vi "Initialize.vi"(8 "error in (no error)":errorcluster, 11 "ChromaPowerSupply in":refnum<class "ChromaPowerSupply.lvclass">) -> (0 "error out":errorcluster, 3 "ChromaPowerSupply out":refnum<class "ChromaPowerSupply.lvclass">)   [LabVIEW 2018, in "AcPwrPlugins.lvlib" / "ChromaPowerSupply.lvclass"]
doc: "This VI establishes communication to the instrument and may provide other functions such as reset the instrument or provide a range check."
uses:
  ChromaPowerSupply.lvclass
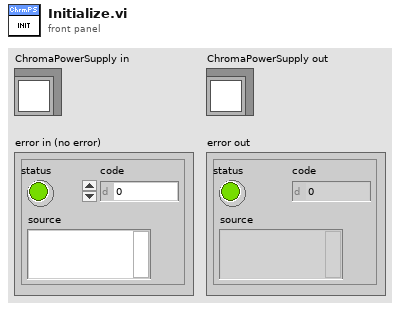
[diagram p1: front panel]
types:
  T1 = cluster{"Handle Connected?":bool, "instrument handle out":refnum<k15>}[]
  T2 = typedef "AcPwrPlugins.lvlib/ChromaPowerSupply.lvclass/Measurements.ctl" = cluster{"Handle":string, "Name":string, "Enabled":bool, "Measurement Value":dbl, "btnMeasFetch":bool, "ProtectionStatusString":string, "Measurement Type":enum16{"Voltage", "Current", "Power"}}[]
  T3 = typedef "AcPwrPlugins.lvlib/ChromaPowerSupply.lvclass/Device(s)Settings.ctl" = cluster{"Phases":cluster{"Handle":string, "Instrument Options":string, "id query (T)":bool, "reset device (T)":bool, "Timing":cluster{"TimingOn":enum16{""}, "Hours":u32, "Minutes":u32, "Seconds":dbl, "CutoffVoltage":dbl}, "Connected":bool, "Output Mode":enum16{"Voltage (DC)", "Current (DC)"}, "Voltage":dbl, "Current":dbl, "High Voltage Limit":dbl, "High Current Limit":dbl, "Power Protect":dbl, "Current Protect":dbl, "Voltage Protect":dbl, "Low Current Limit":dbl, "Low Voltage Limit":dbl, "Current Slew Rate":dbl, "Voltage Slew Rate":dbl, "Current Slew Infinite?":bool}[], "MeasName":string}
  T4 = cluster{"Handle":string, "Instrument Options":string, "id query (T)":bool, "reset device (T)":bool, "Timing":cluster{"TimingOn":enum16{""}, "Hours":u32, "Minutes":u32, "Seconds":dbl, "CutoffVoltage":dbl}, "Connected":bool, "Output Mode":enum16{"Voltage (DC)", "Current (DC)"}, "Voltage":dbl, "Current":dbl, "High Voltage Limit":dbl, "High Current Limit":dbl, "Power Protect":dbl, "Current Protect":dbl, "Voltage Protect":dbl, "Low Current Limit":dbl, "Low Voltage Limit":dbl, "Current Slew Rate":dbl, "Voltage Slew Rate":dbl, "Current Slew Infinite?":bool}[]
  T5 = cluster{"Handle Connected?":bool, "instrument handle out":refnum<k15>}
  T6 = cluster{"Handle":string, "Instrument Options":string, "id query (T)":bool, "reset device (T)":bool, "Timing":cluster{"TimingOn":enum16{""}, "Hours":u32, "Minutes":u32, "Seconds":dbl, "CutoffVoltage":dbl}, "Connected":bool, "Output Mode":enum16{"Voltage (DC)", "Current (DC)"}, "Voltage":dbl, "Current":dbl, "High Voltage Limit":dbl, "High Current Limit":dbl, "Power Protect":dbl, "Current Protect":dbl, "Voltage Protect":dbl, "Low Current Limit":dbl, "Low Voltage Limit":dbl, "Current Slew Rate":dbl, "Voltage Slew Rate":dbl, "Current Slew Infinite?":bool}
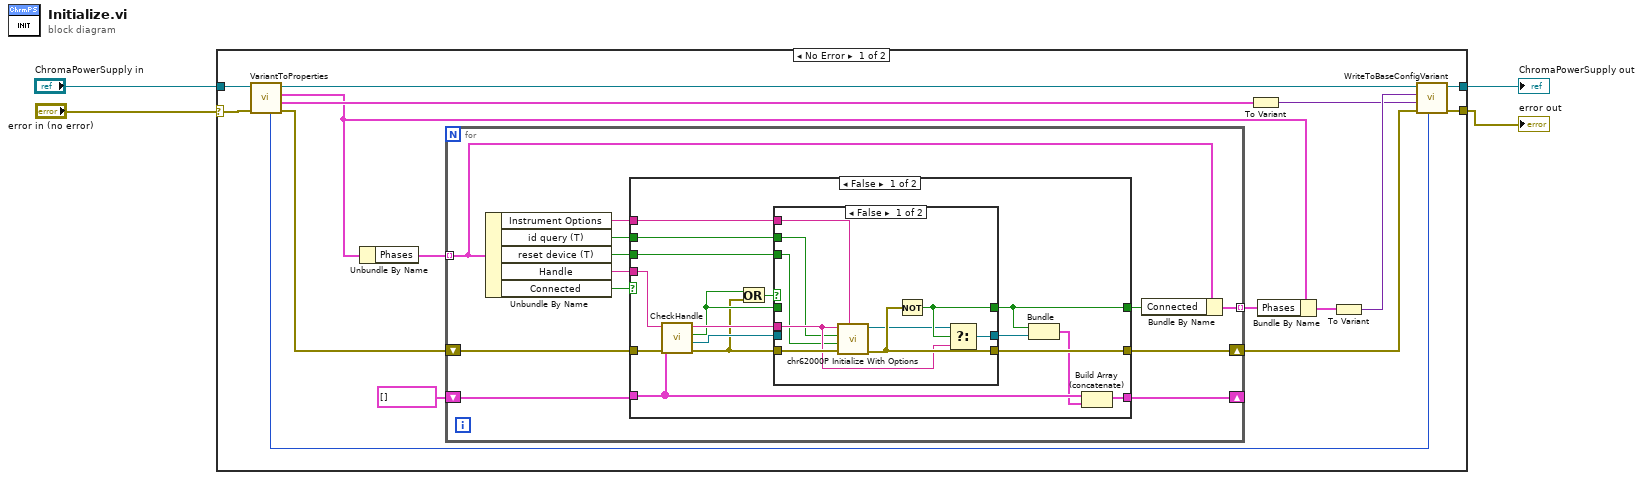
[diagram p0: block diagram]
diagram:
  n1 = case shown="No Error" "error in (no error)" {
    selector: "error in (no error)" -> [w20 w65]
    tunnel: "ChromaPowerSupply in" -> [w10 w64]
    tunnel: [w17 w64] -> w2
    tunnel: [w16 w65] -> w1
    frame No Error {
      n2 = call-dynamic "VariantToProperties.vi"("error in (no error)"=w20, "ChromaPowerSupply in"=w10) -> ("error out"=w19:errorcluster, "Measurements"=w12:T2, "Device Settings"=w7:T3, "ChromaPowerSupply out"=w14:refnum<class "ChromaPowerSupply.lvclass">, "Measurement Refresh Time (ms)"=w11:u32)  [unwired: 5 in]
      n3 = Unbundle By Name(w7) -> ("Phases"=w9:T4)
      n4 = for {
        tunnel: w9 -> [w22] mode=indexing
        shift-right: [w30] -> w15
        shift-left: w19 -> [w31]
        shift-right: [w23] -> _
        shift-left: T1 [] -> [w32]
        tunnel: [w21] -> w8 mode=indexing
        n5 = Unbundle By Name(w22) -> ("Instrument Options"=w26:string, "id query (T)"=w25:bool, "reset device (T)"=w24:bool, "Handle"=w29:string, "Connected"=w28:bool)
        n6 = case shown="False" w28 {
          selector: w28 -> [_ w63]
          tunnel: [w43 w63] -> w27
          tunnel: w29 -> [w48 _]
          tunnel: [w44 w62] -> w30
          tunnel: w31 -> [w37 w62]
          tunnel: w32 -> [w34 w61]
          tunnel: [w46 w61] -> w23
          tunnel: w26 -> [w42 _]
          tunnel: w25 -> [w41 _]
          tunnel: w24 -> [w40 _]
          frame False {
            n7 = call "CheckHandle.vi"("error in (no error)"=w37, "Array"=w34, "Handle In"=w48) -> ("error out"=w35:errorcluster, "instrument handle out"=w39:refnum<k15>, "Handle Connected?"=w36:bool, "Handle Out"=w38:string)  [unwired: 5 in]
            n8 = Or(x=w36, y=w35) -> (x .or. y?=w47:bool)
            n9 = case shown="False" w47 {
              tunnel: [w56 w59] -> w43
              tunnel: w38 -> [w53 _]
              tunnel: w35 -> [w54 w60]
              tunnel: [w55 w60] -> w44
              tunnel: w36 -> [_ w59]
              tunnel: [w57 w58] -> w45
              tunnel: w39 -> [_ w58]
              tunnel: w42 -> [w50 _]
              tunnel: w41 -> [w52 _]
              tunnel: w40 -> [w51 _]
              frame False {
                n10 = call <instrlib>:"chr62000P Initialize With Options.vi"("Option String (\"Simulate=0,RangeCheck=1,QueryInstrStatus=1,Cache=1\")"=w50, "error in (no error)"=w54, "Reset Device (Yes)"=w51, "ID Query (Yes)"=w52, "resource name"=w53) -> ("error out"=w55:errorcluster, "instrument handle out"=w49:refnum<k15>)  [unwired: 5 in]
                n11 = Not(x=w55) -> (.not. x?=w56:bool)
                n12 = Select(t=w49, s=w56, f=w53) -> (s? t:f=w57:refnum<k15>)
              }
              frame True {
              }
            }
            n13 = Bundle("Handle Connected?"=w43, "instrument handle out"=w45) -> (w33:T5)  [unwired: 1 in]
            n14 = Build Array (concatenate)(w34, w33) -> (w46:T1)
          }
          frame True {
          }
        }
        n15 = Bundle By Name(cluster=w22, "Connected"=w27) -> (w21:T6)
      }
      n16 = To Variant(anything=w12) -> (Variant=w13:variant)
      n17 = Bundle By Name(cluster=w7, "Phases"=w8) -> (w6:T3)
      n18 = To Variant(anything=w6) -> (Variant=w18:variant)
      n19 = call-dynamic "WriteToBaseConfigVariant.vi"("Measurement Refresh Time (ms)"=w11, "error in (no error)"=w15, "Meas"=w13, "Config"=w18, "ChromaPowerSupply in"=w14) -> ("error out"=w16:errorcluster, "ChromaPowerSupply out"=w17:refnum<class "ChromaPowerSupply.lvclass">)  [unwired: 5 in]
    }
    frame Error {
    }
  }
  "error out" <- w1
  "ChromaPowerSupply out" <- w2
